vi "FUG_PowerSupply.Reset.vi"(0 "i ref in":refnum<vi>, 5 "error in (no error)":errorcluster) -> (14 "i ref out":refnum<vi>, 19 "error out (no error)":errorcluster)   [LabVIEW 2014, in "FUG_PowerSupply.lvlib"]
doc: "Resets the power supply to its default values and resets the device status."
uses:
  FUG_PowerSupply.lvlib
  CS_Core/CSApplicationBaseClasses/DeviceBase/DeviceBase.deviceState.ctl
  CS_Core/CSApplicationBaseClasses/PSChannelBase/PSChannelBase.lvlib
  CS_Core/CSApplicationBaseClasses/DeviceBase/DeviceBase.lvlib
  CSlibraries/UtilityLib/UtilityLib.lvlib
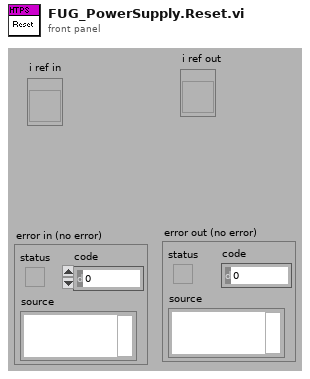
[diagram p1: front panel]
types:
  T1 = typedef "DeviceBase.lvlib/DeviceBase.deviceState.ctl" = i16
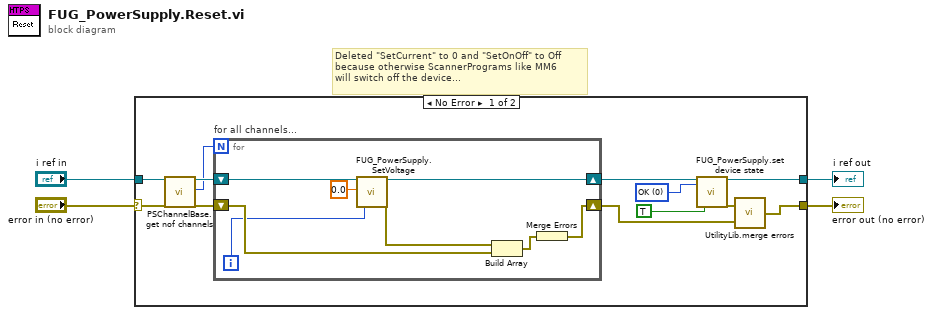
[diagram p0: block diagram]
diagram:
  # "Deleted \"SetCurrent\" to 0 and \"SetOnOff\" to Off\nbecause otherwise ScannerPrograms like MM6\nwill switch off the device..."
  n1 = case shown="No Error" "error in (no error)" {
    selector: "error in (no error)" -> [w15 w26]
    tunnel: "i ref in" -> [w16 w25]
    tunnel: [w6 w25] -> w3
    tunnel: [w7 w26] -> w1
    frame No Error {
      w11 = T1 0 items=["ERROR"=-1, "OK"=0, "NOT_OK"=1] ("deviceState")
      n2 = call "PSChannelBase.get nof channels.vi"("i ref in"=w16, "error in (no error)"=w15) -> ("i ref out"=w13:refnum<vi>, "NofChannels"=w5:i32, "error out"=w14:errorcluster)  [unwired: 15 in]
      n3 = for "for all channels..." {
        N: w5 -> [_]
        shift-right: [w17] -> w12
        shift-left: w13 -> [w18]
        shift-right: [w20] -> w9
        shift-left: w14 -> [w23]
        i -> [w19]
        n4 = call "FUG_PowerSupply.SetVoltage.vi"("i ref in"=w18, "value"=0.0, "channelIndex"=w19) -> ("i ref out"=w17:refnum<vi>, "error out (no error)"=w22:errorcluster)  [unwired: 15 in]
        n5 = Build Array(w22, w23) -> (w21:errorcluster[])
        n6 = Merge Errors(w21) -> (w20:errorcluster)
      }
      n7 = call "FUG_PowerSupply.set device state.vi"("i ref in"=w12, "deviceState"=w11, "mayResetError (FALSE)"=TRUE) -> ("i ref out"=w6:refnum<vi>, "error out"=w8:errorcluster)  [unwired: 14 in, 1 out]
      n8 = call "UtilityLib.merge errors.vi"("error2 (no error)"=w9, "error1 (no error)"=w8) -> ("error out"=w7:errorcluster)
    }
    frame Error {
    }
  }
  "error out (no error)" <- w1
  "i ref out" <- w3
